vi "Check Value Type.vi"(8 "error in (no error)":errorcluster, 11 "Numeric Column in":refnum<class "Numeric Column.lvclass">) -> (0 "error out":errorcluster, 3 "Numeric Column out":refnum<class "Numeric Column.lvclass">)   [LabVIEW 2020, in "Basic Columns.lvlib" / "Numeric Column.lvclass"]
uses:
  Numeric Column.lvclass
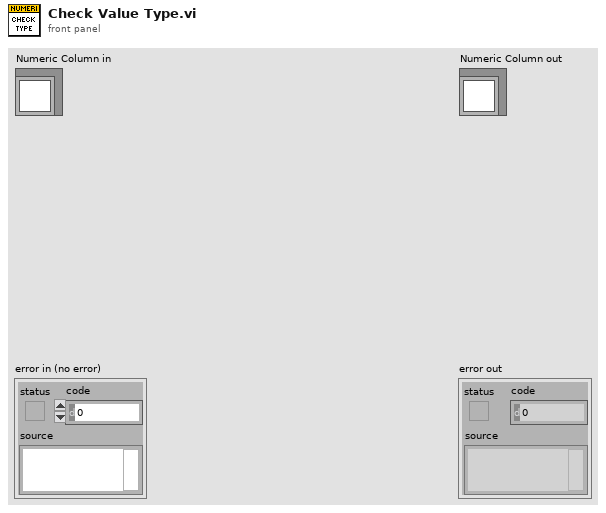
[diagram p1: front panel]
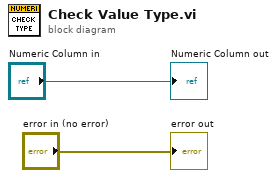
[diagram p0: block diagram]
diagram:
  "error out" <- "error in (no error)"
  "Numeric Column out" <- "Numeric Column in"
